vi "Read Spectrum Analyzer.lvclass.vi"(11 "AM-AM in":refnum<class "AM-AM.lvclass">) -> (2 "Spectrum Analyzer.lvclass":refnum<class "Spectrum Analyzer.lvclass">, 3 "AM-AM out":refnum<class "AM-AM.lvclass">)   [LabVIEW 2020, in "AM-AM.lvclass"]
uses:
  AM-AM.lvclass
  Instruments/Spectrum Analyzer/Spectrum Analyzer.lvclass
  AM-AM.lvclass/AM-AM.ctl
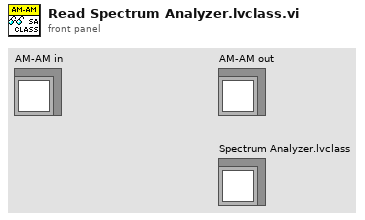
[diagram p1: front panel]
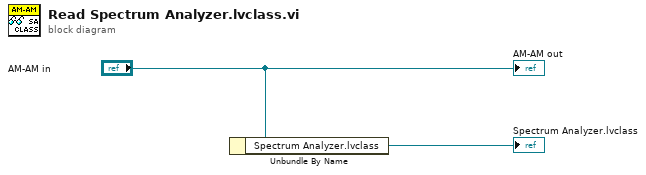
[diagram p0: block diagram]
diagram:
  n1 = Unbundle By Name("AM-AM in") -> ("Spectrum Analyzer.lvclass"=→"Spectrum Analyzer.lvclass":refnum<class "Spectrum Analyzer.lvclass">)
  "AM-AM out" <- "AM-AM in"
